vi "Highlight Line.vi"(7 "Font Color":u32(colorbox)=16711680, 8 "error in (no error)":errorcluster, 10 "Line Number":i32, 11 "String Field In":refnum<vi>) -> (0 "error out":errorcluster, 3 "String Field Out":refnum<vi>)   [LabVIEW 2017]
uses:
  <vilib>/Utility/miscctls.llb/LVSelectionTypeDef.ctl
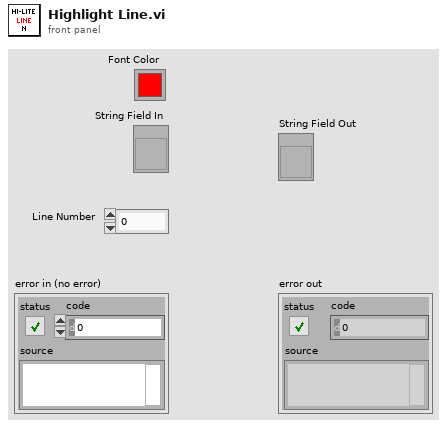
[diagram p1: front panel]
types:
  T1 = typedef "LVSelectionTypeDef.ctl" = cluster{"Selection Start":u32, "Selection End":u32}
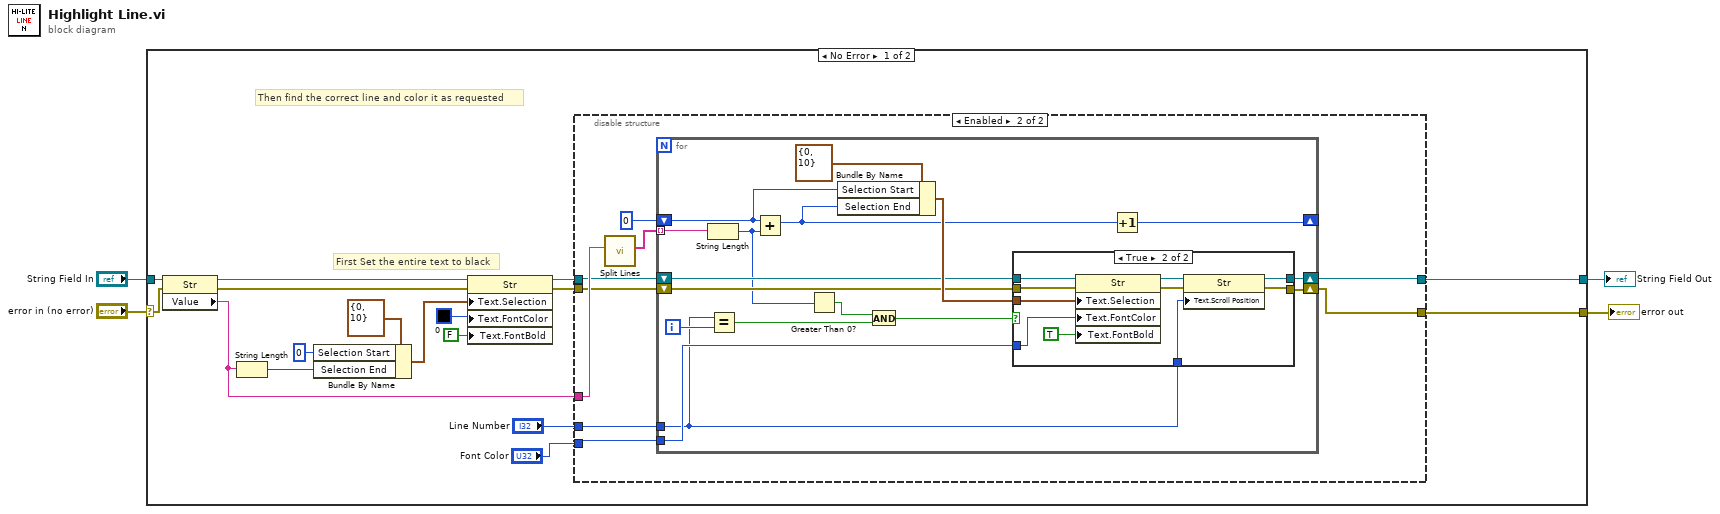
[diagram p0: block diagram]
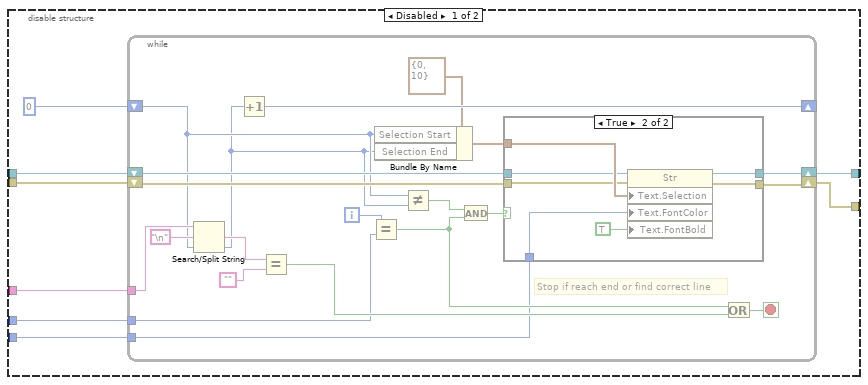
[diagram p2: hidden frame]
diagram:
  n1 = case shown="No Error" "error in (no error)" {
    selector: "error in (no error)" -> [w18 w99]
    tunnel: "String Field In" -> [w21 w98]
    tunnel: [w8 w99] -> w2
    tunnel: [w10 w98] -> w1
    frame No Error {
      # "Then find the correct line and color it as requested"
      # "First Set the entire text to black"
      n2 = property class="Str"(reference=w21, error in=w18) -> (reference out=w20:refnum<vi>, error out=w17:errorcluster, "Value"=w16:string)
      n3 = String Length(string=w16) -> (length=w7:i32)
      n4 = Bundle By Name(cluster=T1 {"Selection Start"=0, "Selection End"=10} ("Text.Selection"), "Selection Start"=u32 0, "Selection End"=w7) -> (w13:T1)
      n5 = property class="Str"(reference=w20, error in=w17, "Text.Selection"=w13, "Text.FontColor"=u32 0 ("Font Color 2"), "Text.FontBold"=FALSE ("Text.Font:Bold")) -> (reference out=w19:refnum<vi>, error out=w9:errorcluster)
      n6 = disable-structure shown="Enabled" {
        disable-tunnel: w19 -> [w28 w65]
        disable-tunnel: w16 -> [w27 w66]
        disable-tunnel: [w26 w61] -> w10
        disable-tunnel: w9 -> [w25 w63]
        disable-tunnel: [w24 w60] -> w8
        disable-tunnel: "Line Number" -> [w23 w64]
        disable-tunnel: "Font Color" -> [w22 w62]
        frame Disabled {
          n7 = while {
            tunnel: w27 -> [w43]
            shift-right: [w50] -> _
            shift-left: 0 -> [w36]
            shift-right: [w44] -> w26
            shift-left: w28 -> [w47]
            shift-right: [w37] -> w24
            shift-left: w25 -> [w38]
            tunnel: w23 -> [w31]
            tunnel: w22 -> [w30]
            i -> [w41]
            stop <- w39 stop-if-true
            # "Stop if reach end or find correct line"
            n8 = Search/Split String(string=w43, search string/char (-)="\n", offset (0)=w36) -> (match + rest of string=w46:string, offset of match=w35:i32)  [unwired: 1 out]
            n9 = Increment(x=w35) -> (x+1=w50:i32)
            n10 = Equal?(x=w46, y="") -> (x = y?=w40:bool)
            n11 = Equal?(x=w41, y=w31) -> (x = y?=w34:bool)
            n12 = Bundle By Name(cluster=T1 {"Selection Start"=0, "Selection End"=10} ("Text.Selection"), "Selection Start"=w36, "Selection End"=w35) -> (w48:T1)
            n13 = Not Equal?(x=w36, y=w35) -> (x != y?=w33:bool)
            n14 = And(x=w33, y=w34) -> (x .and. y?=w32:bool)
            n15 = case shown="True" w32 {
              tunnel: w48 -> [_ w58]
              tunnel: w47 -> [w52 w57]
              tunnel: [w52 w56] -> w44
              tunnel: w38 -> [w51 w55]
              tunnel: [w51 w54] -> w37
              tunnel: w30 -> [_ w53]
              frame False {
              }
              frame True {
                n16 = property class="Str"(reference=w57, error in=w55, "Text.Selection"=w58, "Text.FontColor"=w53, "Text.FontBold"=TRUE ("Text.Font:Bold")) -> (reference out=w56:refnum<vi>, error out=w54:errorcluster)
              }
            }
            n17 = Or(x=w34, y=w40) -> (x .or. y?=w39:bool)
          }
        }
        frame Enabled {
          n18 = call "Split Lines.vi"("String In"=w66) -> ("Lines Out"=w68:string[])  [unwired: 10 in]
          n19 = for {
            tunnel: w68 -> [w84] mode=indexing
            shift-right: [w74] -> _
            shift-left: 0 -> [w79]
            tunnel: w64 -> [w69]
            shift-right: [w77] -> w60
            shift-left: w63 -> [w80]
            shift-right: [w78] -> w61
            shift-left: w65 -> [w81]
            tunnel: w62 -> [w76]
            i -> [w85]
            n20 = String Length(string=w84) -> (length=w72:i32)
            n21 = Equal?(x=w69, y=w85) -> (x = y?=w73:bool)
            n22 = Add(x=w79, y=w72) -> (x+y=w75:i32)
            n23 = Greater Than 0?(x=w72) -> (x > 0?=w71:bool)
            n24 = Bundle By Name(cluster=T1 {"Selection Start"=0, "Selection End"=10} ("Text.Selection"), "Selection Start"=w79, "Selection End"=w75) -> (w83:T1)
            n25 = And(x=w71, y=w73) -> (x .and. y?=w70:bool)
            n26 = case shown="True" w70 {
              tunnel: w83 -> [_ w96]
              tunnel: w81 -> [w87 w95]
              tunnel: [w87 w91] -> w78
              tunnel: w80 -> [w86 w94]
              tunnel: [w86 w89] -> w77
              tunnel: w76 -> [_ w93]
              tunnel: w69 -> [_ w88]
              frame False {
              }
              frame True {
                n27 = property class="Str"(reference=w95, error in=w94, "Text.Selection"=w96, "Text.FontColor"=w93, "Text.FontBold"=TRUE ("Text.Font:Bold")) -> (reference out=w92:refnum<vi>, error out=w90:errorcluster)
                n28 = property class="Str"(reference=w92, error in=w90, "Text.Scroll Position"=w88) -> (reference out=w91:refnum<vi>, error out=w89:errorcluster)
              }
            }
            n29 = Increment(x=w75) -> (x+1=w74:i32)
          }
        }
      }
    }
    frame Error {
    }
  }
  "String Field Out" <- w1
  "error out" <- w2
